vi "Destroy.vi"(8 "ErrorIn":errorcluster, 11 "ReferenceIn":refnum<class "TAFBaseGUI.lvclass">) -> (0 "ErrorOut":errorcluster, 3 "ReferenceOut":refnum<class "TAFBaseGUI.lvclass">)   [LabVIEW 2021, in "TAFBaseGUI.lvclass"]
uses:
  TAFBaseGUI.lvclass
  TAFBaseGUI.lvclass/TAFBaseGUI.ctl
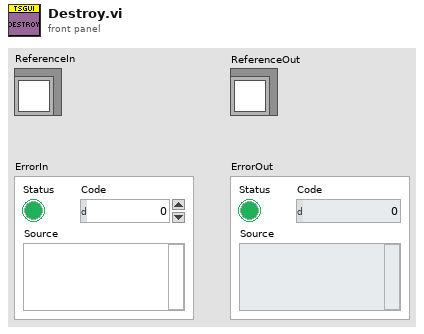
[diagram p1: front panel]
types:
  T1 = typedef "TAFBaseGUI.lvclass/ObjectAttributes.ctl" = cluster{"Name":string, "FPVIRef":refnum<vi>}
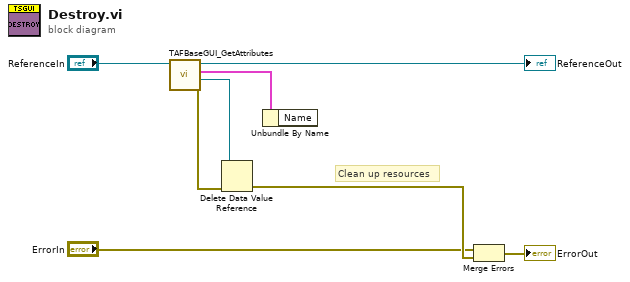
[diagram p0: block diagram]
diagram:
  # "Clean up resources"
  n1 = call "TAFBaseGUI_GetAttributes.vi"("ReferenceIn"="ReferenceIn") -> ("ErrorOut"=w7:errorcluster, "DataRef"=w2:refnum<data-value>, "Data"=w1:T1, "ReferenceOut"=→"ReferenceOut":refnum<class "TAFBaseGUI.lvclass">)  [unwired: 7 in]
  n2 = Delete Data Value Reference(data value reference=w2, error in=w7) -> (error out=w6:errorcluster)  [unwired: 1 out]
  n3 = Unbundle By Name(w1) -> ()  [unwired: 1 out]
  n4 = Merge Errors("ErrorIn", w6) -> (→"ErrorOut":errorcluster)
